vi "Get DS Alert Info.vi"(8 "error in (no error)":errorcluster, 11 "handle":i64) -> (0 "error out":errorcluster)   [LabVIEW 2026, in "MrcLib.lvlib"]
doc: "Return the Alert's status and text referenced by the input handle."
uses:
  MrcLib.lvlib
panel:
  out "isActive?":bool
  out "text":string
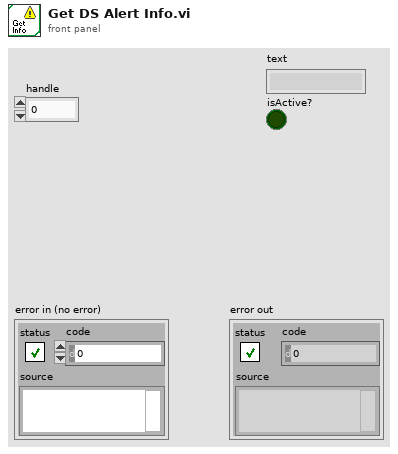
[diagram p1: front panel]
types:
  T1 = typedef "MRC String.ctl" = cluster{"pointer":u64, "length":u64}
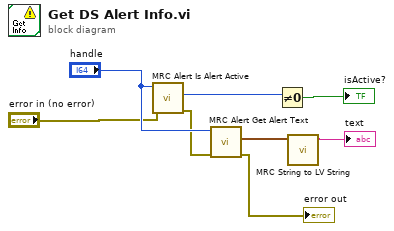
[diagram p0: block diagram]
diagram:
  n1 = call "MRC Alert Is Alert Active.vi"("error in (no error)"="error in (no error)", "handle"="handle") -> ("error out"=w3:errorcluster, "isActive"=w5:u8)  [unwired: 8 in]
  n2 = call "MRC Alert Get Alert Text.vi"("error in (no error)"=w3, "handle"="handle") -> ("error out"=→"error out":errorcluster, "text"=w7:T1)  [unwired: 8 in]
  n3 = Not Equal To 0?(x=w5) -> (x != 0?=→"isActive?":bool)
  n4 = call "MRC String to LV String.vi"("MRC String"=w7) -> ("LV String"=→"text":string)  [unwired: 10 in]
